vi "bundleScanParameters.vi"(8 "error in (no error)":errorcluster, 9 "Zoom":dbl[](array[numeric]), 10 "xyzNormalizedCoordinates":T1={"XYZ Start"=[{"X"=0.0, "Y"=0.0, "Z"=0.0}], "XYZ Stop"=[]}, 11 "AOL_Globals":T2={"Imaging Protocol"=enum."AOL Z-Stack", "Number of POI"=0, "Number of Miniscans"=0, "Number of Trials"=0, "Number of Cycles "=0, "# Averaged Frames"=0, "Laser power (%)"=0, "Pockels (V)"=0.0, "Acquisition Length (sec)"=0.0, "Fill time (us)"=0.0, "POI Dwell time (us)"=0.0, "Miniscan Dwell time per pixel (us)"=0.0, "PMT 1"=0.0, "PMT 2"=0.0, "Back Apperture (mA)"=200.0, "Frame Size"=0, "Center Frequency"=0.0, "Field of View (um)"=175.0, "Field of View (norm)"=0.0, "DwellTime (us)"=0.0, "Ref Dwell Time (us)"=0.0, "Wavelength (nm)"=0.0, "Zoom"=0.0, "AOL Z"=0.0, "AOL Mode"=enum."Raster", "GridXY"=0.0, "GridZ"=0.0, "TriggerPeriod (sec)"=0.0, "Number of Pixels in Miniscan"=0, "Experiment folder path"=path "", "X centre"=0.0, "Y centre"=0.0, "Angle (degrees)"=0.0, "Angle Xs (degrees)"=0.0, "Angle Ys (degrees)"=0.0, "Plane Mode"=0, "Threshold"=[], "Regenerate Chirps"=FALSE, "Rectangle ROI length (pixels)"=0, "Rectangle ROI height (pixels)"=0, "AOD fill"=4900, "StartupDelay"=0, "Samples Wait after Trigger"=5080, "Slip Cycle"=600000, "Add Cycle"=TRUE, "Functional Mode"=enum."Point", "Z Start"=0.0, "Z Stop"=0.0, "# Planes"=0, "Total Pixels"=0, "Variable Miniscan Pixels"=[], "Use Variable Length"=FALSE, "Use Variable Resolution"=FALSE, "Laser power (%) at Z Start"=0, "Laser power (%) at Z Stop"=0, "Ref Z Step"=0} {"Angle Ys (degrees)" format="%#.6g"; "Angle Xs (degrees)" format="%#.6g"; "Plane Mode" items=["XY Plane", "XZ Plane", "YZ Plane", "arbitraryplane"]; "Frame Size" items=["100X100"=100, "128X128"=128, "200X200"=200, "256X256"=256, "512X512"=512, "1024x1024"=1024, "2048x2048"=2048]; "Back Apperture (mA)" format="%#.6g"; "Pockels (V)" format="%#.6g"; "PMT 2" format="%#.6g"; "PMT 1" format="%#.6g"; "Angle (degrees)" format="%#.6g"; "POI Dwell time (us)" format="%#.6g"}) -> (0 "error out":errorcluster, 1 "xyzImageStopNormalised":dbl[][](array[numeric]), 2 "xyzImageStartNormalised":dbl[][](array[numeric]), 3 "scanVariables":dbl[][](array[numeric]), 4 "XYZ Array size":i32[](array[numeric]), 5 "Number of Miniscans":u16, 7 "Use Variable Length":bool)   [LabVIEW 2020]
uses:
  Typedefs/Controls/AOL_Globals.ctl
  Typedefs/Imaging Protocols enum.ctl
  Typedefs/Frame Size.ctl
  Typedefs/AOL modes.ctl
  Typedefs/Plane Mode.ctl
  Typedefs/Functional Mode.ctl
  Global Variables/General Globals.vi
  Global Variables/gl_UI Ctrl Refs.vi
panel:
  in  "Bypass with this manual value 2":bool caption="Bypass with this manual value"
  in  "Field of View":dbl
  out "size":i32
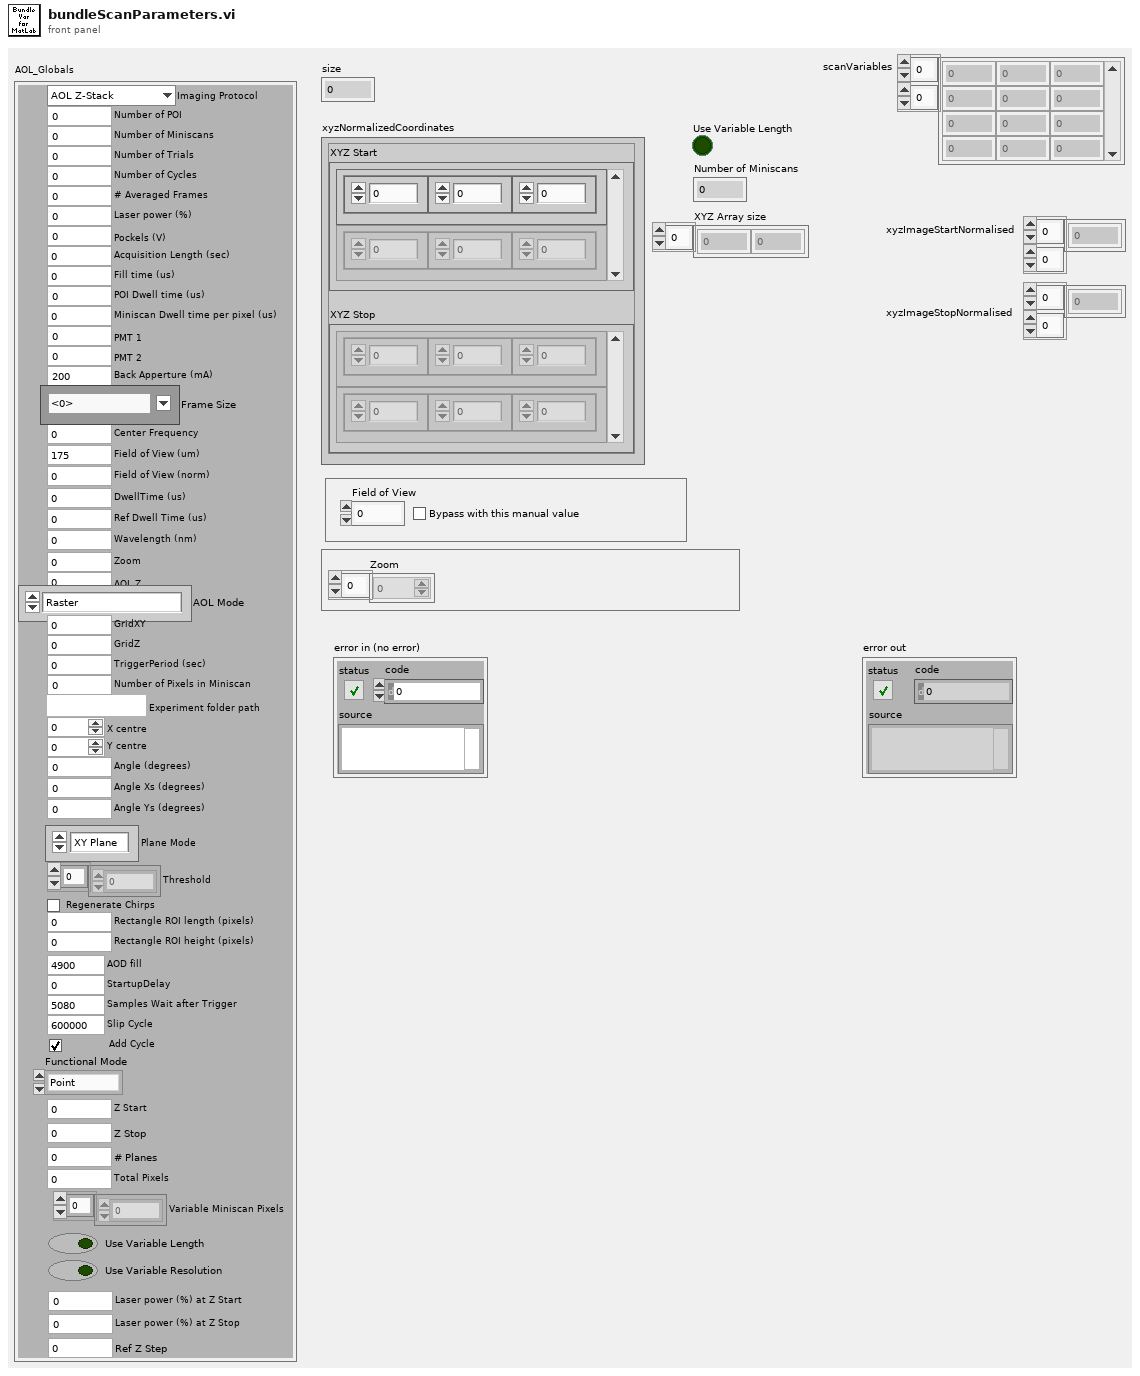
[diagram p1: front panel]
types:
  T1 = cluster{"XYZ Start":cluster{"X":sgl, "Y":sgl, "Z":sgl}[], "XYZ Stop":cluster{"X":sgl, "Y":sgl, "Z":sgl}[]}
  T2 = typedef "AOL_Globals.ctl" = cluster{"Imaging Protocol":T3, "Number of POI":u16, "Number of Miniscans":u16, "Number of Trials":u16, "Number of Cycles ":u64, "# Averaged Frames":u16, "Laser power (%)":u8, "Pockels (V)":dbl, "Acquisition Length (sec)":dbl, "Fill time (us)":dbl, "POI Dwell time (us)":dbl, "Miniscan Dwell time per pixel (us)":dbl, "PMT 1":dbl, "PMT 2":dbl, "Back Apperture (mA)":dbl, "Frame Size":T4, "Center Frequency":dbl, "Field of View (um)":dbl, "Field of View (norm)":dbl, "DwellTime (us)":dbl, "Ref Dwell Time (us)":dbl, "Wavelength (nm)":dbl, "Zoom":dbl, "AOL Z":dbl, "AOL Mode":T5, "GridXY":dbl, "GridZ":dbl, "TriggerPeriod (sec)":dbl, "Number of Pixels in Miniscan":u16, "Experiment folder path":path, "X centre":dbl, "Y centre":dbl, "Angle (degrees)":dbl, "Angle Xs (degrees)":dbl, "Angle Ys (degrees)":dbl, "Plane Mode":T6, "Threshold":u16[], "Regenerate Chirps":bool, "Rectangle ROI length (pixels)":u16, "Rectangle ROI height (pixels)":u16, "AOD fill":u16, "StartupDelay":i32, "Samples Wait after Trigger":u16, "Slip Cycle":u32, "Add Cycle":bool, "Functional Mode":T7, "Z Start":dbl, "Z Stop":dbl, "# Planes":i32, "Total Pixels":i32, "Variable Miniscan Pixels":u16[], "Use Variable Length":bool, "Use Variable Resolution":bool, "Laser power (%) at Z Start":u8, "Laser power (%) at Z Stop":u8, "Ref Z Step":i8}
  T3 = typedef "Imaging Protocols enum.ctl" = enum16{"AOL Z-Stack", "Motor Z Stack", "Parameter Sweep", "Functional Acquisition", "Single Plane Acquisition", "Volume Acquisition", "Live Imaging", "Live Plane Imaging", "Live Volume Imaging"}
  T4 = typedef "Frame Size.ctl" = u16
  T5 = typedef "AOL modes.ctl" = enum16{"Raster", "Structural", "Pointing", "Mini Scan", "Alignment"}
  T6 = typedef "Plane Mode.ctl" = u16
  T7 = typedef "Functional Mode.ctl" = enum16{"Point", "Line", "Patch", "Plane", "Volume"}
  T8 = typedef "UI ctrl refs cluster.ctl" = cluster{"Top level VI path":path, "Top level VI ref":refnum<vi>, "User menu ref":refnum<k9>, "Sub Panel control":refnum<vi>, "Imaging Param Tab":refnum<vi>, "Occurrence-Start drivers":refnum<k4>, "Occurrence-Speed logging initialised":refnum<k4>, "Occurrence-XYZ stage initialised":refnum<k4>, "Exit button":refnum<vi>, "Status ind":refnum<vi>, "Set as origin":refnum<vi>, "Speed Logging":refnum<vi>, "Time Lapse":refnum<vi>, "Live Imaging":refnum<vi>, "AOL Z Stack":refnum<vi>, "Motor Z Stack":refnum<vi>, "Funct Acq button":refnum<vi>, "Hard Shutter":refnum<vi>, "Virtual Shutter":refnum<vi>, "Laser Power":refnum<vi>, "AOL Mode":refnum<vi>, "Frame Size":refnum<vi>, "Field of View":refnum<vi>, "Dwell Time":refnum<vi>, "Zoom":refnum<vi>, "AOL Z":refnum<vi>, "Objective":refnum<vi>, "Axis":refnum<vi>, "Paths & Names":refnum<vi>, "Experiment folder path (ind.)":refnum<vi>, "Last State (Ind.)":refnum<vi>, "Averages":refnum<vi>, "Angle (degrees)":refnum<vi>, "X centre":refnum<vi>, "Y centre":refnum<vi>, "Plane Mode":refnum<vi>, "# Planes":refnum<vi>, "Z Start":refnum<vi>, "Z Stop":refnum<vi>, "Z Step":refnum<vi>, "PMT 1":refnum<vi>, "PMT 2":refnum<vi>, "Stage XYZ Position":refnum<vi>, "Pockels@Z Start":refnum<vi>, "Pockels@Z Stop":refnum<vi>, "Obtain Z Start":refnum<vi>, "Obtain Z Stop":refnum<vi>, "Live stim.trig.period":refnum<vi>, "Live stim.trig.enable":refnum<vi>, "Movement Correction":refnum<vi>, "Load Reference Image":refnum<vi>, "XY Stage Move":refnum<vi>, "MovCor Cluster":refnum<vi>, "RefDAQParam":refnum<vi>, "Funct. Acq. Pockels Modulation":refnum<vi>, "Ref Laser Power":refnum<vi>, "Enable Video Recording":refnum<vi>, "Video Record-Live Imaging":refnum<vi>, "Video Record-Funct acq":refnum<vi>, "Reference Source":refnum<vi>, "AOL Z-stack Chirps Ready (ind)":refnum<vi>, "Target time between mov.cor. ref triggers (ms)":refnum<vi>, "Funct. Acq. Ref frame save":refnum<vi>, "Tracking button":refnum<vi>, "Show ref plots window":refnum<vi>, "Center freq ind (nm)":refnum<vi>, "Pickup mode (ind)":refnum<vi>, "Logging queue (ind)":refnum<vi>, "Back aperture power (ind.)":refnum<vi>, "Power after objective (ind.)":refnum<vi>, "Switch user":refnum<vi>, "Ls1 Conn. Status":refnum<vi>, "Ls1Tuning Status":refnum<vi>, "Ls1 Faults":refnum<vi>, "Ls1 Connection":refnum<vi>, "Ls1 Mode":refnum<vi>, "Ls1 POWER [mW]":refnum<vi>, "Ls1Shutter":refnum<vi>, "Ls1 Wavelength":refnum<vi>, "Ls1 Note":refnum<vi>, "Ls1 Confirm Wav":refnum<vi>, "Ls1 PreChrp Prism1":refnum<vi>, "Ls1 PreChrp Prism2":refnum<vi>, "Ls1 wav top Ind":refnum<vi>, "Ls1 power top Ind":refnum<vi>, "Ls1 Pump peak Hold":refnum<vi>, "Ls1 Status Ind":refnum<vi>, "Ls1 wav cancel":refnum<vi>, "Experiment Type":refnum<vi>, "Biology Information":refnum<vi>, "Camera recording status":refnum<vi>, "Optimise Obj. Pos.":refnum<vi>}
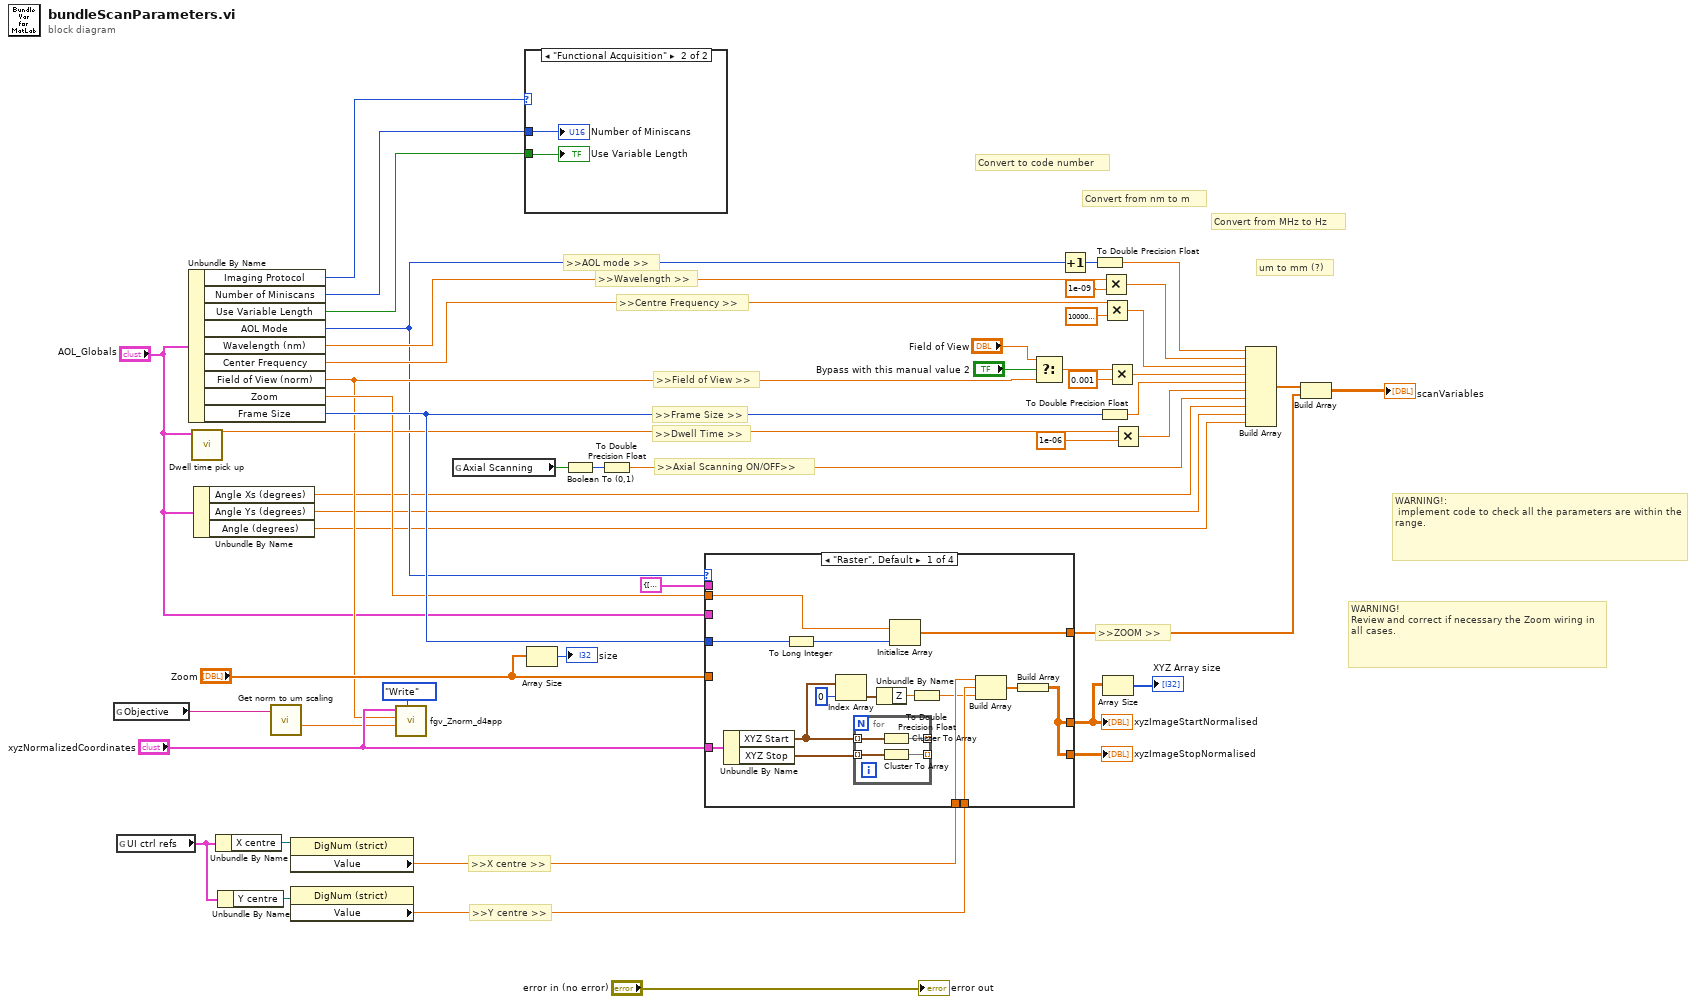
[diagram p0: block diagram]
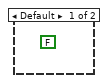
[diagram p2: hidden frame]
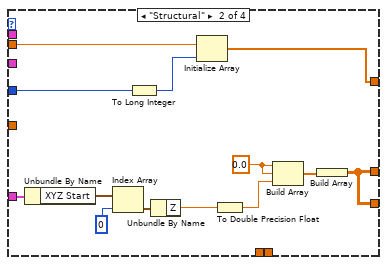
[diagram p3: hidden frame]
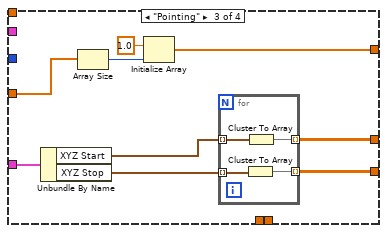
[diagram p4: hidden frame]
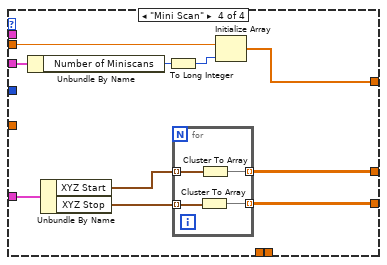
[diagram p5: hidden frame]
diagram:
  # ">>Y centre >>"
  # ">>X centre >>"
  # ">>ZOOM >>"
  # ">>Axial Scanning ON/OFF>>"
  # ">>Dwell Time >>"
  # ">>Frame Size >>"
  # "um to mm (?)"
  # ">>Field of View >>"
  # "Convert from MHz to Hz"
  # "Convert from nm to m"
  # "Convert to code number"
  # ">>Centre Frequency >>"
  # ">>Wavelength >>"
  # ">>AOL mode >>"
  # "WARNING!\nReview and correct if necessary the Zoom wiring in all cases."
  # "WARNING!:\n implement code to check all the parameters are within the range."
  n1 = global read "General Globals.vi" "Objective"() -> (w19:string)
  n2 = global read "gl_UI Ctrl Refs.vi" "UI ctrl refs"() -> (w12:T8)
  n3 = Unbundle By Name("AOL_Globals") -> ("Imaging Protocol"=w5:T3, "Number of Miniscans"=w6:u16, "Use Variable Length"=w7:bool, "AOL Mode"=w9:T5, "Wavelength (nm)"=w50:dbl, "Center Frequency"=w43:dbl, "Field of View (norm)"=w15:dbl, "Zoom"=w33:dbl, "Frame Size"=w34:T4)
  n4 = call "Dwell time pick up.vi"("AOL_Globals"="AOL_Globals") -> ("Dwell time (us)"=w29:dbl)  [unwired: 10 in]
  n5 = Unbundle By Name("AOL_Globals") -> ("Angle Xs (degrees)"=w3:dbl, "Angle Ys (degrees)"=w2:dbl, "Angle (degrees)"=w1:dbl)
  n6 = Unbundle By Name(w12) -> ("X centre"=w14:refnum<vi>)
  n7 = Unbundle By Name(w12) -> ("Y centre"=w13:refnum<vi>)
  n8 = call "Get norm to um scaling .vi"("Current Objective"=w19) -> ("Z_norm to um_scaling"=w16:dbl)  [unwired: 7 in, 3 out]
  n9 = property class="DigNum (strict)"(reference=w14) -> ("Value"=w11:dbl)  [unwired: 1 in, 2 out]
  n10 = property class="DigNum (strict)"(reference=w13) -> ("Value"=w10:dbl)  [unwired: 1 in, 2 out]
  n11 = call "fgv_Znorm_d4app.vi"("Function"=enum16{"Idle", "Write", "Read"}."Write", "Znorm_um_Scaling"=w16, "acceptance angle"=w15, "xyzNormalizedCoordinates"="xyzNormalizedCoordinates") -> ()  [unwired: 5 in, 3 out]
  n12 = global read "General Globals.vi" "Axial Scanning"() -> (w20:bool)
  n13 = case shown="\"Functional Acquisition\"" w5 {
    tunnel: w7 -> [_ w51]
    tunnel: w6 -> [_ w52]
    frame Default {
      (unwired) FALSE ("Use Variable Length")
    }
    frame "Functional Acquisition" {
      "Use Variable Length" <- w51
      "Number of Miniscans" <- w52
    }
  }
  n14 = Array Size(array="Zoom") -> (size(s)=→"size":i32)
  n15 = Boolean To (0,1)(Boolean=w20) -> (0, 1=w23:i16)
  n16 = To Double Precision Float(number=w23) -> (double precision float=w22:dbl)
  n17 = case shown="\"Raster\", Default" w9 {
    tunnel: "xyzNormalizedCoordinates" -> [w67 w74 w93 w107]
    tunnel: T1 {"XYZ Start"=[{"X"=0.0, "Y"=0.0, "Z"=0.0}], "XYZ Stop"=[]} ("xyzNormalizedCoordinates") -> [_ _ _ _]
    tunnel: [w60 w77 w91 w101] -> w31
    tunnel: [w60 w77 w85 w98] -> w37
    tunnel: w34 -> [w63 w83 _ _]
    tunnel: [w65 w84 w87 w103] -> w24
    tunnel: w33 -> [w64 w81 _ w104]
    tunnel: "Zoom" -> [_ _ w88 _]
    tunnel: "AOL_Globals" -> [_ _ _ w106]
    tunnel: w11 -> [w59 _ _ _]
    tunnel: w10 -> [w58 _ _ _]
    frame "Raster", Default {
      n18 = Unbundle By Name(w67) -> ("XYZ Start"=w56:cluster{"X":sgl, "Y":sgl, "Z":sgl}[], "XYZ Stop"=w66:cluster{"X":sgl, "Y":sgl, "Z":sgl}[])
      n19 = To Long Integer(number=w63) -> (32bit integer=w62:i32)
      n20 = Index Array(array=w56, index=0) -> (element=w55:cluster{"X":sgl, "Y":sgl, "Z":sgl})
      n21 = for {
        tunnel: w56 -> [w71] mode=indexing
        tunnel: [w70] -> _ mode=indexing
        tunnel: w66 -> [w69] mode=indexing
        tunnel: [w68] -> _ mode=indexing
        n22 = Cluster To Array(cluster=w71) -> (array=w70:sgl[])
        n23 = Cluster To Array(cluster=w69) -> (array=w68:sgl[])
      }
      n24 = Unbundle By Name(w55) -> ("Z"=w54:sgl)
      n25 = Initialize Array(w64, w62) -> (w65:dbl[])
      n26 = To Double Precision Float(number=w54) -> (double precision float=w53:dbl)
      n27 = Build Array(w59, w58, w53) -> (w61:dbl[])
      n28 = Build Array(w61) -> (w60:dbl[][])
    }
    frame "Structural" {
      w79 = 0.0 ("element")
      n29 = Unbundle By Name(w74) -> ("XYZ Start"=w73:cluster{"X":sgl, "Y":sgl, "Z":sgl}[])
      n30 = Index Array(array=w73, index=0) -> (element=w76:cluster{"X":sgl, "Y":sgl, "Z":sgl})
      n31 = To Long Integer(number=w83) -> (32bit integer=w82:i32)
      n32 = Unbundle By Name(w76) -> ("Z"=w72:sgl)
      n33 = Initialize Array(w81, w82) -> (w84:dbl[])
      n34 = To Double Precision Float(number=w72) -> (double precision float=w78:dbl)
      n35 = Build Array(w79, w79, w78) -> (w80:dbl[])
      n36 = Build Array(w80) -> (w77:dbl[][])
    }
    frame "Pointing" {
      n37 = Unbundle By Name(w93) -> ("XYZ Start"=w92:cluster{"X":sgl, "Y":sgl, "Z":sgl}[], "XYZ Stop"=w86:cluster{"X":sgl, "Y":sgl, "Z":sgl}[])
      n38 = Array Size(array=w88) -> (size(s)=w90:i32)
      n39 = Initialize Array(1.0 ("element"), w90) -> (w87:dbl[])
      n40 = for {
        tunnel: w92 -> [w97] mode=indexing
        tunnel: [w96] -> w91 mode=indexing
        tunnel: w86 -> [w95] mode=indexing
        tunnel: [w94] -> w85 mode=indexing
        n41 = Cluster To Array(cluster=w95) -> (array=w94:sgl[])
        n42 = Cluster To Array(cluster=w97) -> (array=w96:sgl[])
      }
    }
    frame "Mini Scan" {
      n43 = Unbundle By Name(w106) -> ("Number of Miniscans"=w105:u16)
      n44 = Unbundle By Name(w107) -> ("XYZ Start"=w100:cluster{"X":sgl, "Y":sgl, "Z":sgl}[], "XYZ Stop"=w99:cluster{"X":sgl, "Y":sgl, "Z":sgl}[])
      n45 = To Long Integer(number=w105) -> (32bit integer=w102:i32)
      n46 = for {
        tunnel: w100 -> [w111] mode=indexing
        tunnel: [w110] -> w101 mode=indexing
        tunnel: w99 -> [w109] mode=indexing
        tunnel: [w108] -> w98 mode=indexing
        n47 = Cluster To Array(cluster=w109) -> (array=w108:sgl[])
        n48 = Cluster To Array(cluster=w111) -> (array=w110:sgl[])
      }
      n49 = Initialize Array(w104, w102) -> (w103:dbl[])
    }
  }
  "xyzImageStartNormalised" <- w31
  "xyzImageStopNormalised" <- w37
  n50 = Select(t="Field of View", s="Bypass with this manual value 2", f=w15) -> (s? t:f=w28:dbl)
  n51 = Increment(x=w9) -> (x+1=w21:T5)
  n52 = To Double Precision Float(number=w21) -> (double precision float=w49:dbl)
  n53 = To Double Precision Float(number=w34) -> (double precision float=w47:dbl)
  n54 = Multiply(x=w50, y=1e-09) -> (x*y=w46:dbl)
  n55 = Multiply(x=w43, y=1000000.0) -> (x*y=w44:dbl)
  n56 = Array Size(array=w31) -> (size(s)=→"XYZ Array size":i32[])
  n57 = Multiply(x=w28, y=0.001) -> (x*y=w39:dbl)
  n58 = Multiply(x=w29, y=1e-06) -> (x*y=w41:dbl)
  n59 = Build Array(w49, w46, w44, w39, w47, w41, w22, w3, w2, w1) -> (w36:dbl[])
  n60 = Build Array(w36, w24) -> (→"scanVariables":dbl[][])
  "error out" <- "error in (no error)"
